vi "DataHandler64.vi"(0 "Data Cycles Per Buffer":i32, 1 "Rx Packet Byte size":i32=67, 3 "data out":string) -> (2 "Unscaled Data":u16[](array[numeric]), 5 "Scaled Buffer Array":sgl[](array[numeric]), 6 "Rx Byte Array":u8[](array[numeric]), 7 "Rx Byte Array (no headers)":u8[](array[numeric]), 9 "Data":sgl[][](array[numeric]))   [LabVIEW 2021]
panel:
  out "Removed Headers":u8[][](array[numeric])
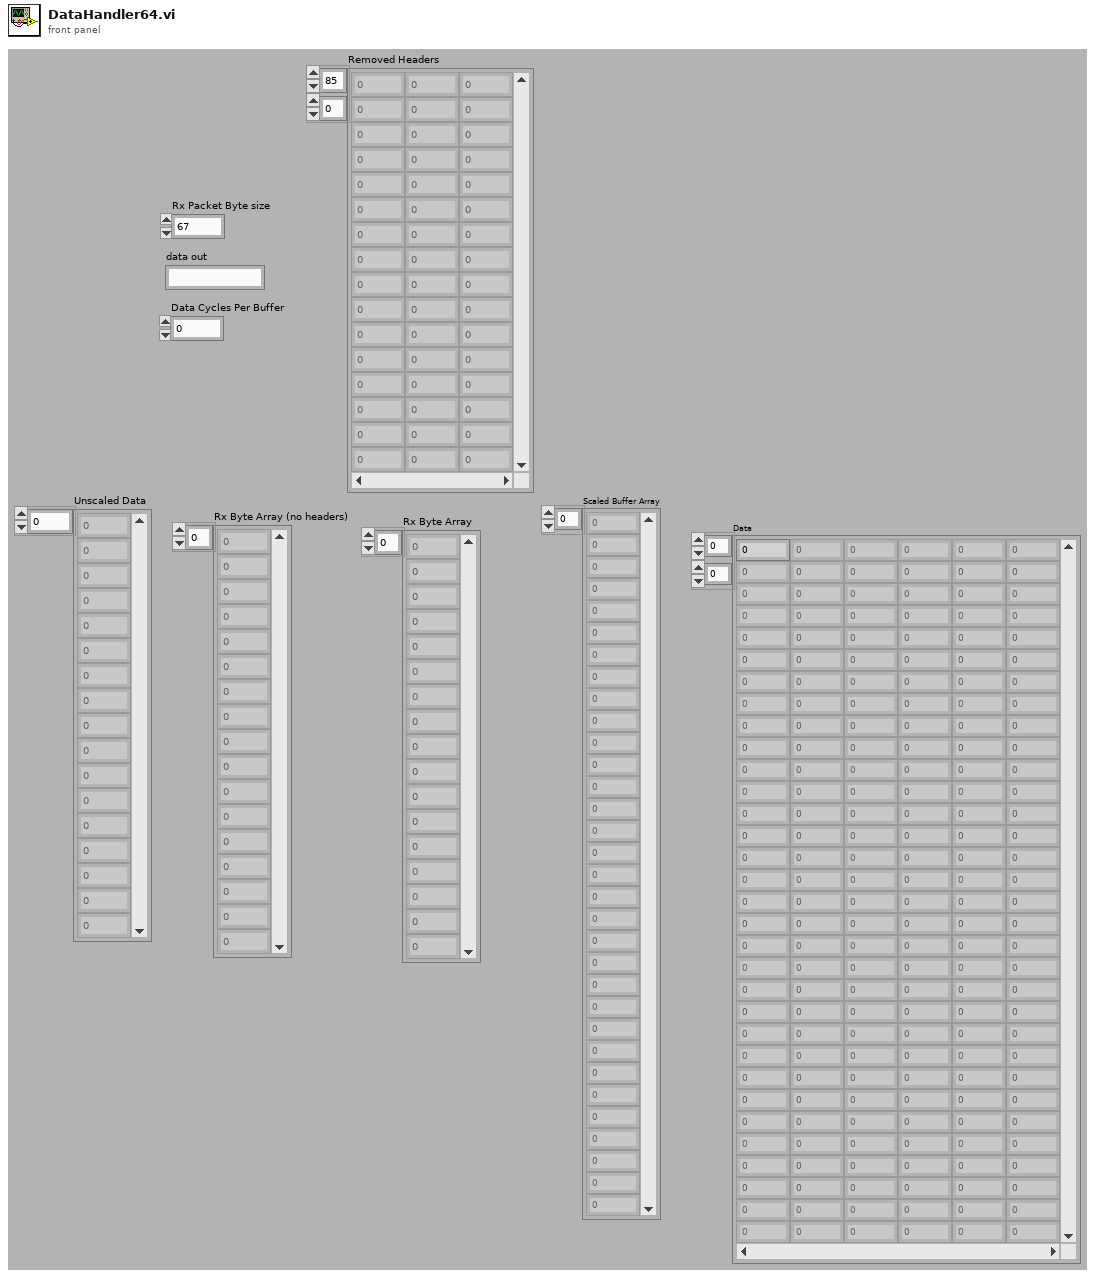
[diagram p1: front panel]
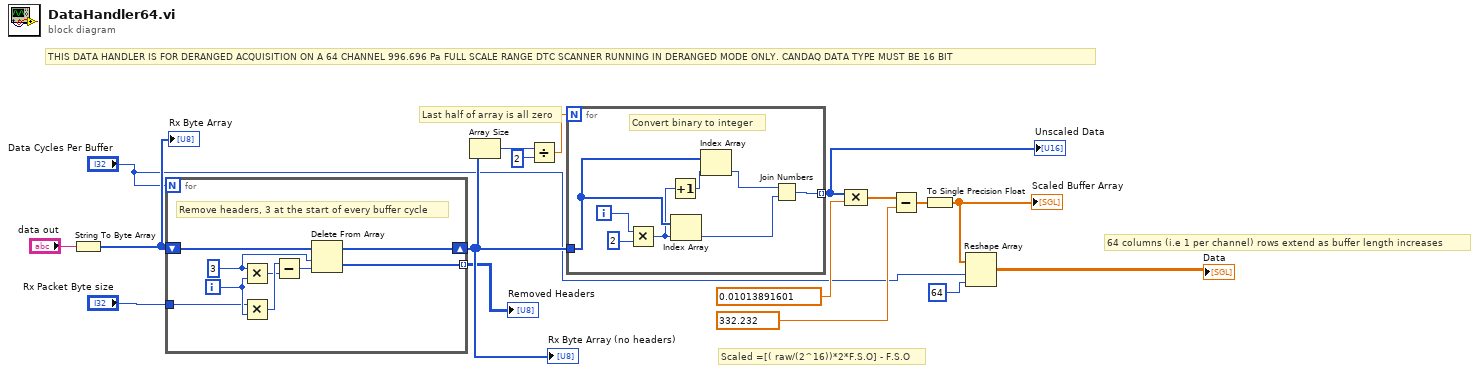
[diagram p0: block diagram]
diagram:
  # "Last half of array is all zero"
  # "64 columns (i.e 1 per channel) rows extend as buffer length increases"
  # "Scaled =[( raw/(2^16))*2*F.S.O] - F.S.O"
  # "THIS DATA HANDLER IS FOR DERANGED ACQUISITION ON A 64 CHANNEL 996.696 Pa FULL SCALE RANGE DTC SCANNER RUNNING IN DERANGED MODE ONLY. CANDAQ DATA TYPE MUST BE 16 BIT"
  n1 = String To Byte Array(string="data out") -> (unsigned byte array=w11:u8[])
  "Rx Byte Array" <- w11
  n2 = for {
    N: "Data Cycles Per Buffer" -> [_]
    shift-right: [w26] -> w10
    shift-left: w11 -> [w25]
    tunnel: "Rx Packet Byte size" -> [w19]
    tunnel: [w18] -> w7 mode=indexing
    i -> [w22]
    w23 = 3 ("length")
    # "Remove headers, 3 at the start of every buffer cycle"
    n3 = Multiply(x=w23, y=w22) -> (x*y=w21:i32)
    n4 = Multiply(x=w19, y=w22) -> (x*y=w24:i32)
    n5 = Subtract(x=w24, y=w21) -> (x-y=w20:i32)
    n6 = Delete From Array(array=w25, length=w23, index=w20) -> (deleted portion=w18:u8[], array with subset deleted=w26:u8[])
  }
  "Rx Byte Array (no headers)" <- w10
  "Removed Headers" <- w7
  n7 = Array Size(array=w10) -> (size(s)=w12:i32)
  n8 = Divide(x=w12, y=2) -> (x/y=w14:dbl)
  n9 = for {
    N: w14 -> [_]
    tunnel: w10 -> [w34]
    tunnel: [w33] -> w2 mode=indexing
    i -> [w32]
    # "Convert binary to integer"
    n10 = Multiply(x=w32, y=2) -> (x*y=w29:i32)
    n11 = Increment(x=w29) -> (x+1=w30:i32)
    n12 = Index Array(array=w34, index=w29) -> (element=w27:u8)
    n13 = Index Array(array=w34, index=w30) -> (element=w28:u8)
    n14 = Join Numbers(hi=w28, lo=w27) -> ((hi.lo)=w33:u16)
  }
  "Unscaled Data" <- w2
  n15 = Compound Arithmetic op=MULTIPLY(w2, 0.01013891601 ("x")) -> (w16:dbl[])
  n16 = Subtract(x=w16, y=332.232 ("x")) -> (x-y=w6:dbl[])
  n17 = To Single Precision Float(number=w6) -> (single precision float=w3:sgl[])
  "Scaled Buffer Array" <- w3
  n18 = Reshape Array(w3, "Data Cycles Per Buffer", 64 ("dimension size")) -> (→"Data":sgl[][])
